vi "Get and Check PID Parameters.vi"(8 "error in (no error)":errorcluster, 11 "MulticolumnListbox in":refnum<vi>) -> (0 "error out":errorcluster, 2 "PID Parameters":T1(array[cluster]), 3 "MulticolumnListbox out":refnum<vi>)   [LabVIEW 2015, in "PID Control Workspace Tool.lvlib"]
uses:
  PID Control Workspace Tool.lvlib
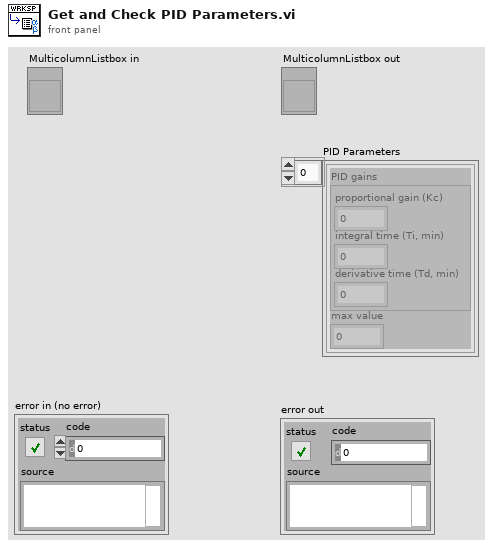
[diagram p1: front panel]
types:
  T1 = cluster{"PID gains":cluster{"proportional gain (Kc)":dbl, "integral time (Ti, min)":dbl, "derivative time (Td, min)":dbl}, "max value":dbl}[]
  T2 = cluster{"PID gains":cluster{"proportional gain (Kc)":dbl, "integral time (Ti, min)":dbl, "derivative time (Td, min)":dbl}, "max value":dbl}
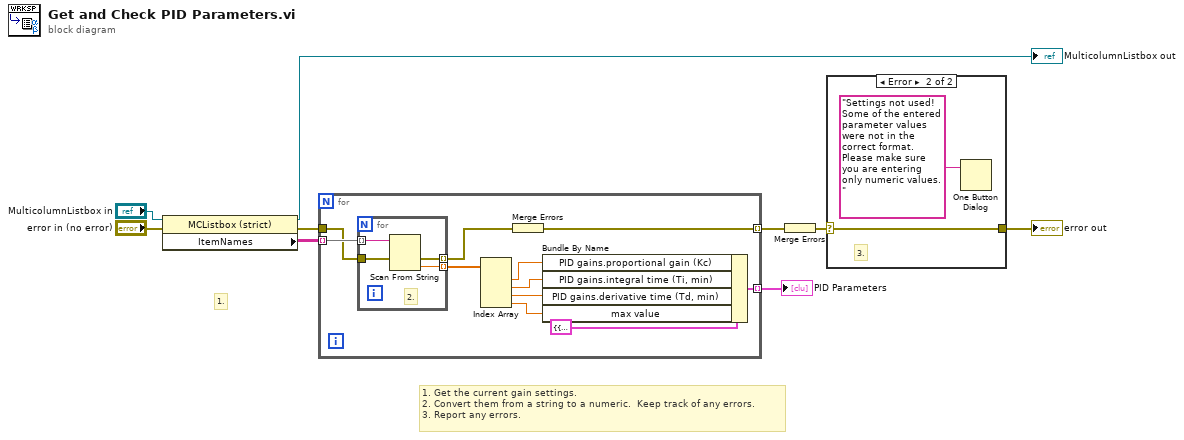
[diagram p0: block diagram]
diagram:
  # "1. Get the current gain settings.\n2. Convert them from a string to a numeric.  Keep track of any errors.\n3. Report any errors."
  # "1."
  n1 = property on="Property Node" class="MCListbox (strict)"(reference="MulticolumnListbox in", error in="error in (no error)") -> (reference out=→"MulticolumnListbox out":refnum<vi>, error out=w6:errorcluster, "ItemNames"=w8:string[][])
  n2 = for {
    tunnel: w8 -> [w20] mode=indexing
    tunnel: [w13] -> w9 mode=indexing
    tunnel: w6 -> [w11]
    tunnel: [w10] -> w5 mode=indexing
    n3 = for {
      tunnel: w20 -> [w24] mode=indexing
      tunnel: [w23] -> w19 mode=indexing
      tunnel: [w22] -> w12 mode=indexing
      tunnel: w11 -> [w21]
      # "2."
      n4 = Scan From String(input string=w24, error in=w21) -> (error out=w22:errorcluster, output 1=w23:dbl)  [unwired: 3 in, 2 out]
    }
    n5 = Index Array(array=w19) -> (element #1=w17:dbl, element #2=w16:dbl, element #3=w15:dbl, element #4=w14:dbl)  [unwired: 4 in]
    n6 = Merge Errors(w12) -> (w10:errorcluster)
    n7 = Bundle By Name(cluster=T2 {"PID gains"={"proportional gain (Kc)"=0.0, "integral time (Ti, min)"=0.0, "derivative time (Td, min)"=0.0}, "max value"=0.0} ("gain schedule"), "PID gains.proportional gain (Kc)"=w17, "PID gains.integral time (Ti, min)"=w16, "PID gains.derivative time (Td, min)"=w15, "max value"=w14) -> (w13:T2)
  }
  "PID Parameters" <- w9
  n8 = Merge Errors(w5) -> (w4:errorcluster)
  n9 = case shown="Error" w4 {
    selector: w4 -> [w25 w27]
    tunnel: [w25 w27] -> w3
    frame No Error {
    }
    frame Error {
      # "3."
      n10 = One Button Dialog(message="Settings not used!  Some of the entered parameter values were not in the correct format.  Please make sure you are entering only numeric values.") -> ()  [unwired: 1 in, 1 out]
    }
  }
  "error out" <- w3
